vi "Log Messages set.vi"(10 "SerialNumber":string, 11 "Message set":T1[](array[typedef])) -> ()   [LabVIEW 2025]
uses:
  Controls/Control Message set.ctl
  Communication Handle/API/Commands.ctl
  <vilib>/Utility/file.llb/Write Delimited Spreadsheet (string).vi
panel:
  out "error out":errorcluster
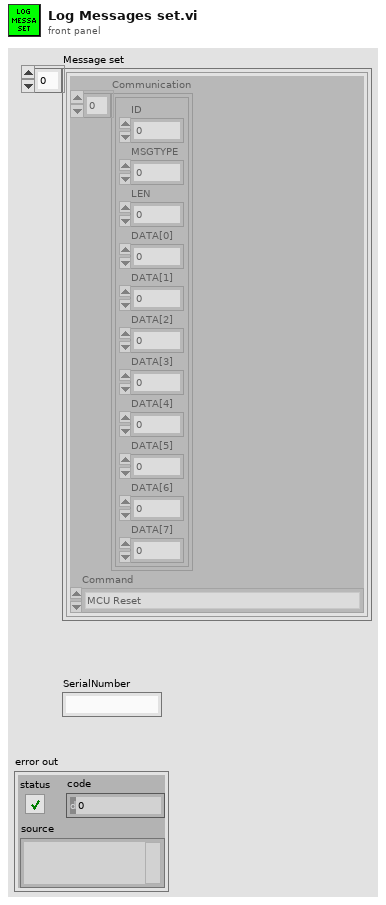
[diagram p1: front panel]
types:
  T1 = typedef "Control Message set.ctl" = cluster{"Communication":cluster{"ID":u32, "MSGTYPE":u8, "LEN":u8, "DATA[0]":u8, "DATA[1]":u8, "DATA[2]":u8, "DATA[3]":u8, "DATA[4]":u8, "DATA[5]":u8, "DATA[6]":u8, "DATA[7]":u8}[], "Command":T2}
  T2 = typedef "Commands.ctl" = enum16{"Nexteer connect", "Write Polarity", "Write BEMF", "Write Torque Scale Sensors T1", "Write Torque Scale Sensors T2", "Trim HW Torque Sensors T1", "Trim HW Torque Sensors T2", "Read HW Torque Trim Performed Sensors T1", "Read HW Torque Trim Performed Sensors T2", "Write EOL Offset values to defaults", "Write EOL Gain values to defaults", "Write Serial Number", "Write Hardware Part Number", "Write EPS Serial Number", "Read MEC Counter", "MCU Reset", "Read System State", "Read First Motor Position", "Manufacturing Diagnostic Defeat", "Perform Current Offset ", "Current Offset Status", "Enable Engine Run", "Perform Current Gain ", "Current Gain Status", "Disable Torque Ramp Down ", "Disable Engine Run", "Set Vehicle Speed Override", "Read Offset Values Using FD F5", "Read Gain Values Using FD F4", "Clear Nexteer NTCs", "Read Second Motor Position", "Read ECU Software ID", "Read Internal Software Version", "Read Bootloader ID", "Read Bootloader Software Version", "Read Calibration Release 0", "Read Calibration Release 1", "Read Calibration Release 2", "Read Temperature  ", "Battery Voltage  ", "Read Motor Angle 0", "Read Motor Angle 1 ", "Set Motor Torque Command ", "Read Motor Current   ", "Stop Motor Torque Command", "Read NTCs", "Read Serial Number", "Read HW Part Number", "Read Polarity", "Set NVM Access Defeat", "Read Software Release", "Read Software Build Date", "Write Single Inverter Hardware value", "Write Dual Inverter Hardware value", "Read Single Inverter HW Value", "Read Dual Inverter HW Value", "Write MEC Counter FE", "Write MEC Counter FF", "Read BEMF", "Read Torque 1 FDB6", "Read Torque 2 FDB7", "Read Torque Trim 1 FDB4", "Read Torque Trim 2 FDB5", "Write Torque Trim 1 FDB4", "Write Torque Trim 2 FDB5", "XCP connect", "Read HW Torque T1", "Read HW Torque T2", "Read Motor Speed "}
  T3 = cluster{"ID":u32, "MSGTYPE":u8, "LEN":u8, "DATA[0]":u8, "DATA[1]":u8, "DATA[2]":u8, "DATA[3]":u8, "DATA[4]":u8, "DATA[5]":u8, "DATA[6]":u8, "DATA[7]":u8}[]
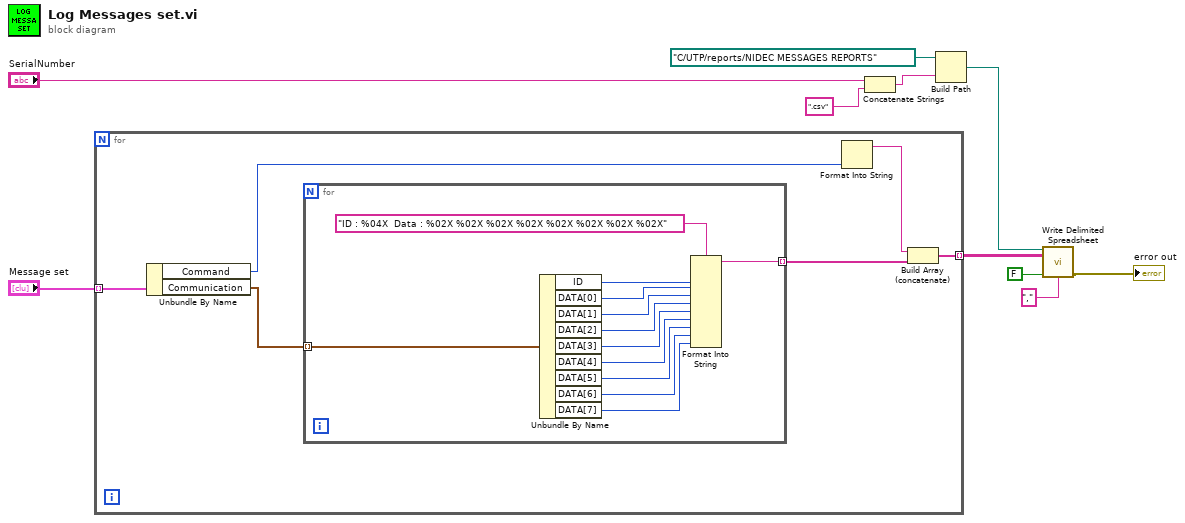
[diagram p0: block diagram]
diagram:
  n1 = for {
    tunnel: "Message set" -> [w16] mode=indexing
    tunnel: [w11] -> w7 mode=indexing
    n2 = Unbundle By Name(w16) -> ("Command"=w15:T2, "Communication"=w14:T3)
    n3 = for {
      tunnel: w14 -> [w28] mode=indexing
      tunnel: [w17] -> w12 mode=indexing
      n4 = Unbundle By Name(w28) -> ("ID"=w27:u32, "DATA[0]"=w26:u8, "DATA[1]"=w25:u8, "DATA[2]"=w24:u8, "DATA[3]"=w23:u8, "DATA[4]"=w22:u8, "DATA[5]"=w21:u8, "DATA[6]"=w20:u8, "DATA[7]"=w19:u8)
      n5 = Format Into String(format string="ID : %04X  Data : %02X %02X %02X %02X %02X %02X %02X %02X", w27, w26, w25, w24, w23, w22, w21, w20, w19) -> (resulting string=w17:string)  [unwired: 2 in, 1 out]
    }
    n6 = Format Into String(w15) -> (resulting string=w13:string)  [unwired: 3 in, 1 out]
    n7 = Build Array (concatenate)(w13, w12) -> (w11:string[])
  }
  n8 = Concatenate Strings("SerialNumber", ".csv" ("string")) -> (w5:string)
  n9 = Build Path(base path=path "C:/UTP/reports/NIDEC MESSAGES REPORTS" ("file path (dialog if empty)"), name or relative path=w5) -> (appended path=w2:path)
  n10 = call-poly <vilib>:"Write Delimited Spreadsheet.vi"("file path (dialog if empty)"=w2, "2D data"=w7, "append to file? (new file:F)"=FALSE, "delimiter (\\t)"="," ("delimiter (\\t)")) -> ("error out"=→"error out":errorcluster)  [unwired: 10 in, 1 out]
